vi "ACP Fetch.vi"(0 "RFmx Handle In":refnum<k21>, 1 "Selector String":string, 11 "error in (no error)":errorcluster) -> (4 "RFmx Handle Out":refnum<k21>, 6 "ACP Results":T1, 15 "error out":errorcluster)   [LabVIEW 2018, in "RFmxLTE.lvlib"]
uses:
  RFmxLTE.lvlib
  Typedefs/ACP Results.ctl
  Typedefs/ACP Offset Results.ctl
  Typedefs/ACP CC Results.ctl
  <vilib>/RFmx/LTE/mx/RFmxLTE.llb/RFmxLTE ACP Fetch Component Carrier Measurement (Array).vi
  <vilib>/RFmx/LTE/mx/RFmxLTE.llb/RFmxLTE ACP Fetch Offset Measurement (Array).vi
  <resource>/objmgr/RFmxLTE.rc
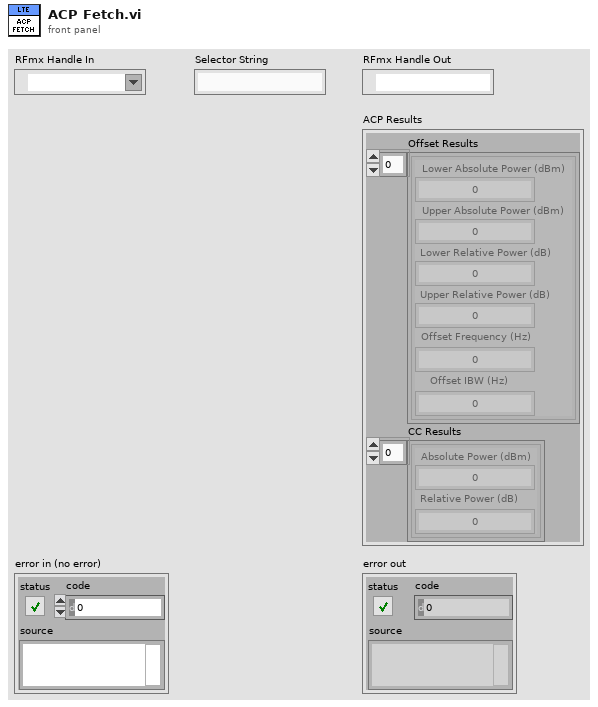
[diagram p1: front panel]
types:
  T1 = typedef "RFmxLTE.lvlib/ACP Results.ctl" = cluster{"Offset Results":T2[], "CC Results":T3[]}
  T2 = typedef "RFmxLTE.lvlib/ACP Offset Results.ctl" = cluster{"Lower Absolute Power (dBm)":dbl, "Upper Absolute Power (dBm)":dbl, "Lower Relative Power (dB)":dbl, "Upper Relative Power (dB)":dbl, "Offset Frequency (Hz)":dbl, "Offset IBW (Hz)":dbl}
  T3 = typedef "RFmxLTE.lvlib/ACP CC Results.ctl" = cluster{"Absolute Power (dBm)":dbl, "Relative Power (dB)":dbl}
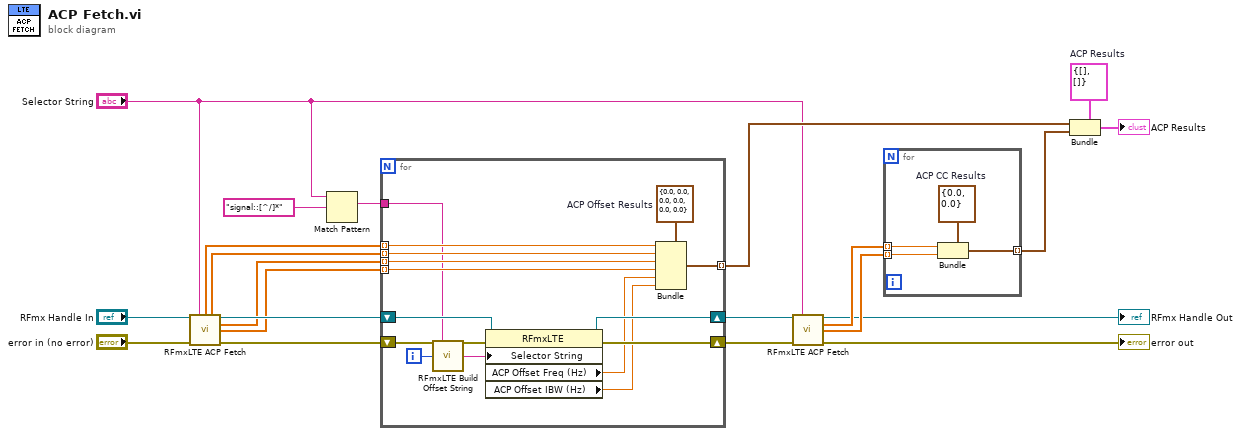
[diagram p0: block diagram]
diagram:
  w21 = T1 {"Offset Results"=[], "CC Results"=[]}  # ACP Results
  n1 = call-poly <vilib>:"RFmxLTE ACP Fetch.vi"("Instrument Handle In"="RFmx Handle In", "Selector String"="Selector String", "error in (no error)"="error in (no error)") -> ("Lower Absolute Power (dBm)"=w13:dbl[], "Upper Absolute Power (dBm)"=w12:dbl[], "Instrument Handle Out"=w15:refnum<k21>, "Lower Relative Power (dB)"=w11:dbl[], "Upper Relative Power (dB)"=w10:dbl[], "error out"=w14:errorcluster)  [unwired: 7 in]
  n2 = Match Pattern(string="Selector String", regular expression="signal::[^/]*") -> (match substring=w8:string)  [unwired: 1 in, 3 out]
  n3 = for {
    shift-right: [w34] -> w7
    shift-left: w15 -> [w28]
    shift-right: [w35] -> w6
    shift-left: w14 -> [w27]
    tunnel: [w30] -> w18 mode=indexing
    tunnel: w13 -> [w26] mode=indexing
    tunnel: w12 -> [w25] mode=indexing
    tunnel: w11 -> [w24] mode=indexing
    tunnel: w10 -> [w23] mode=indexing
    tunnel: w8 -> [w22]
    i -> [w36]
    w33 = T2 {"Lower Absolute Power (dBm)"=0.0, "Upper Absolute Power (dBm)"=0.0, "Lower Relative Power (dB)"=0.0, "Upper Relative Power (dB)"=0.0, "Offset Frequency (Hz)"=0.0, "Offset IBW (Hz)"=0.0}  # ACP Offset Results
    n4 = call <vilib>:"RFmxLTE Build Offset String.vi"("Selector String"=w22, "Offset Number"=w36) -> ("Selector String Out"=w29:string)  [unwired: 13 in]
    n5 = property class="RFmxLTE"(reference=w28, error in=w27, "Selector String"=w29) -> (reference out=w34:refnum<k21>, error out=w35:errorcluster, "ACP Offset Freq (Hz)"=w31:dbl, "ACP Offset IBW (Hz)"=w32:dbl)
    n6 = Bundle(cluster=w33, "Lower Absolute Power (dBm)"=w26, "Upper Absolute Power (dBm)"=w25, "Lower Relative Power (dB)"=w24, "Upper Relative Power (dB)"=w23, "Offset Frequency (Hz)"=w31, "Offset IBW (Hz)"=w32) -> (w30:T2)
  }
  n7 = call-poly <vilib>:"RFmxLTE ACP Fetch.vi"("Instrument Handle In"=w7, "Selector String"="Selector String", "error in (no error)"=w6) -> ("Instrument Handle Out"=→"RFmx Handle Out":refnum<k21>, "Absolute Power (dBm)"=w4:dbl[], "Relative Power (dB)"=w3:dbl[], "error out"=→"error out":errorcluster)  [unwired: 9 in]
  n8 = for {
    tunnel: [w40] -> w19 mode=indexing
    tunnel: w4 -> [w38] mode=indexing
    tunnel: w3 -> [w37] mode=indexing
    w39 = T3 {"Absolute Power (dBm)"=0.0, "Relative Power (dB)"=0.0}  # ACP CC Results
    n9 = Bundle(cluster=w39, "Absolute Power (dBm)"=w38, "Relative Power (dB)"=w37) -> (w40:T3)
  }
  n10 = Bundle(cluster=w21, "Offset Results"=w18, "CC Results"=w19) -> (→"ACP Results":T1)
